vi "GlobalVariableDemo.vi"() -> ()   [LabVIEW 2019]
uses:
  LEDSOnGlobal.vi
panel:
  out "LED 2":bool
  out "LED 1":bool
  in  "Boolean":bool
  # "LED 1 On"
  # "LED 2 On"
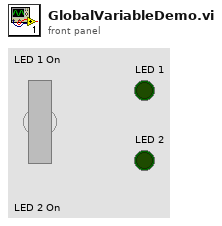
[diagram p1: front panel]
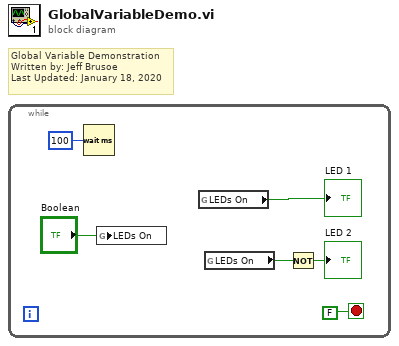
[diagram p0: block diagram]
diagram:
  # "Global Variable Demonstration\nWritten by: Jeff Brusoe\nLast Updated: January 18, 2020"
  n1 = while {
    stop <- FALSE stop-if-true
    n2 = Wait (ms)(milliseconds to wait=u32 100) -> ()  [unwired: 1 out]
    n3 = global write "LEDSOnGlobal.vi" "LEDs On"("Boolean") -> ()
    n4 = global read "LEDSOnGlobal.vi" "LEDs On"() -> (→"LED 1":bool)
    n5 = global read "LEDSOnGlobal.vi" "LEDs On"() -> (w1:bool)
    n6 = Not(x=w1) -> (.not. x?=→"LED 2":bool)
  }
